vi "Boiler Main - UI.vi"() -> ()   [LabVIEW 2012]
panel:
  in  "App Stop":bool
  in  "Boiler Simulation Controls":T1 {"Flame Sensor Value (%)" scale=0.0..100.0}
  in  "Boiler Controls":T2 {"Fuel Control Valve Position (% Open)" scale=0.0..100.0}
  out "Boiler Status Indicators":T3 {"Time Count (s)" format="%.2f"}
  # "On"
  # "Off"
  # "Closed"
  # "Open"
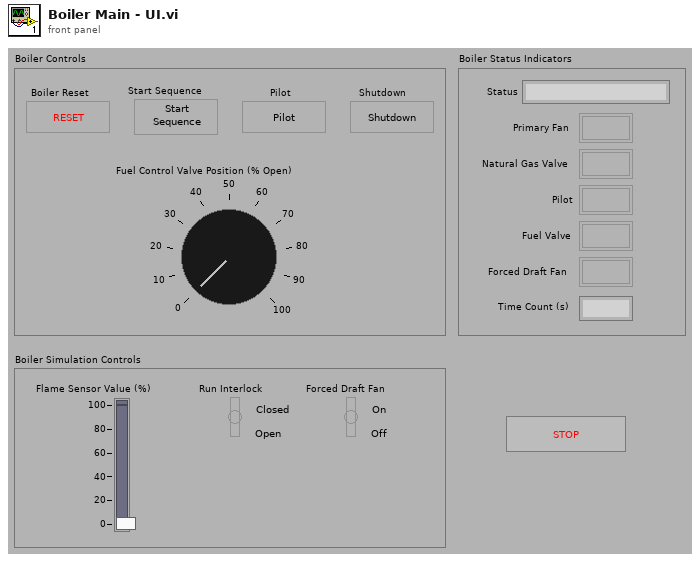
[diagram p1: front panel]
types:
  T1 = cluster{"Flame Sensor Value (%)":dbl, "Run Interlock":bool, "Forced Draft Fan":bool}
  T2 = cluster{"Shutdown":bool, "Pilot Button":bool, "Start Sequence":bool, "Boiler Reset":bool, "Fuel Control Valve Position (% Open)":dbl}
  T3 = cluster{"Time Count (s)":dbl, "Status":string, "Forced Draft Fan":bool, "Fuel Valve":bool, "Pilot Indicator":bool, "Natural Gas Valve":bool, "Primary Fan":bool}
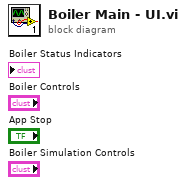
[diagram p0: block diagram]
diagram:
